vi "TDMS Optimizations (SubVI).vi"(11 "Optimizations in":T1) -> (3 "Optimizations":T1)   [LabVIEW 2023]
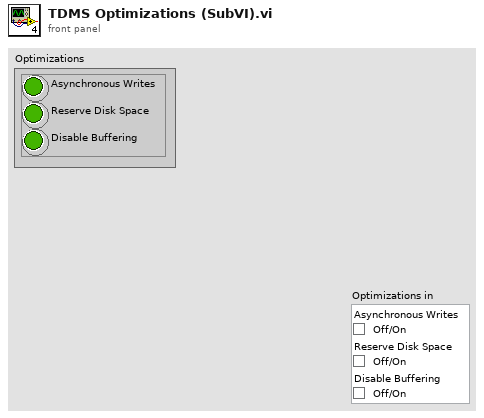
[diagram p1: front panel]
types:
  T1 = cluster{"Asynchronous Writes":bool, "Reserve Disk Space":bool, "Disable Buffering":bool}
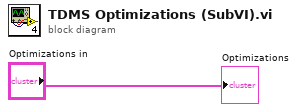
[diagram p0: block diagram]
diagram:
  "Optimizations" <- "Optimizations in"
